vi "Launch Disaster.vi"(11 "VI Path":path) -> ()   [LabVIEW 2019]
doc: "Launch a disaster VI. The disaster VI being called must have a VI ref input, used for the VI ref corresponding to the top-most block diagram."
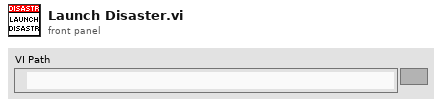
[diagram p1: front panel]
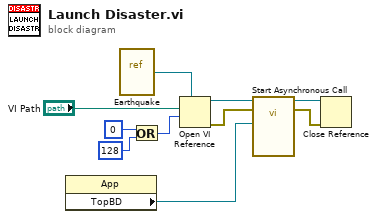
[diagram p0: block diagram]
diagram:
  n1 = property class="App"() -> ("TopBD"=w9:refnum<vi>)  [unwired: 2 in, 2 out]
  n2 = vi-ref "Earthquake.vi"() -> (w7:refnum<vi>)
  n3 = Or(x=0 ("options"), y=128 ("options")) -> (x .or. y?=w3:i32)
  n4 = Open VI Reference(type specifier VI Refnum (for type only)=w7, vi path="VI Path", options=w3) -> (vi reference=w8:refnum<vi>, error out=w6:errorcluster)  [unwired: 3 in]
  n5 = call-by-ref "Start Asynchronous Call"(reference=w8, error in=w6, "VI Ref"=w9) -> (reference out=w2:refnum<vi>, error out=w1:errorcluster)  [unwired: 11 in]
  n6 = Close Reference(reference=w2, error in (no error)=w1) -> ()  [unwired: 1 out]
